vi "NumIntegrate_Rkf45impl_Ax_Bu_K.vi"(4 "MaxTruncError":dbl, 5 "A":T1, 6 "dT_Remaining":dbl, 7 "B":T1, 8 "InitialH":dbl, 9 "K":T1, 10 "U":T1, 11 "X":T1) -> (1 "IterationCount":i32, 2 "H":dbl, 3 "NewX":T1)   [LabVIEW 2019, in "Trajectory_Library.lvlib"]
doc: "Creates a new LINEAR SYSTEM data cluster with the specified values. \n\n\nInputs: \n - XXX -- XXX.\n\nOutputs:\n - XXX -- XXX."
uses:
  Trajectory_Library.lvlib
  <vilib>/Analysis/Matrix/Datatypes/RealMatrix.ctl
  <vilib>/Analysis/_algsub.llb/Matrix Norm Type.ctl
  <vilib>/Analysis/_algsub.llb/Real Matrix Norm.vi
  <vilib>/Analysis/Matrix/Numeric/Multiply/Multiply - RM,R.vi
  <vilib>/Analysis/Matrix/Numeric/Add/Add - RM,RM.vi
  <vilib>/Analysis/Matrix/NI_Matrix.lvlib
  <vilib>/Analysis/NI_AALPro.lvlib
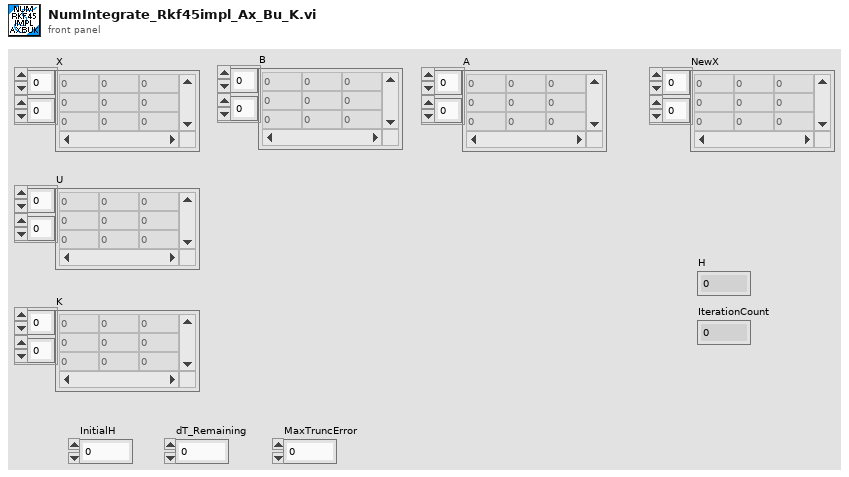
[diagram p1: front panel]
types:
  T1 = typedef "NI_Matrix.lvlib/RealMatrix.ctl" = dbl[][]
  T2 = typedef "NI_AALPro.lvlib/Matrix Norm Type.ctl" = i32
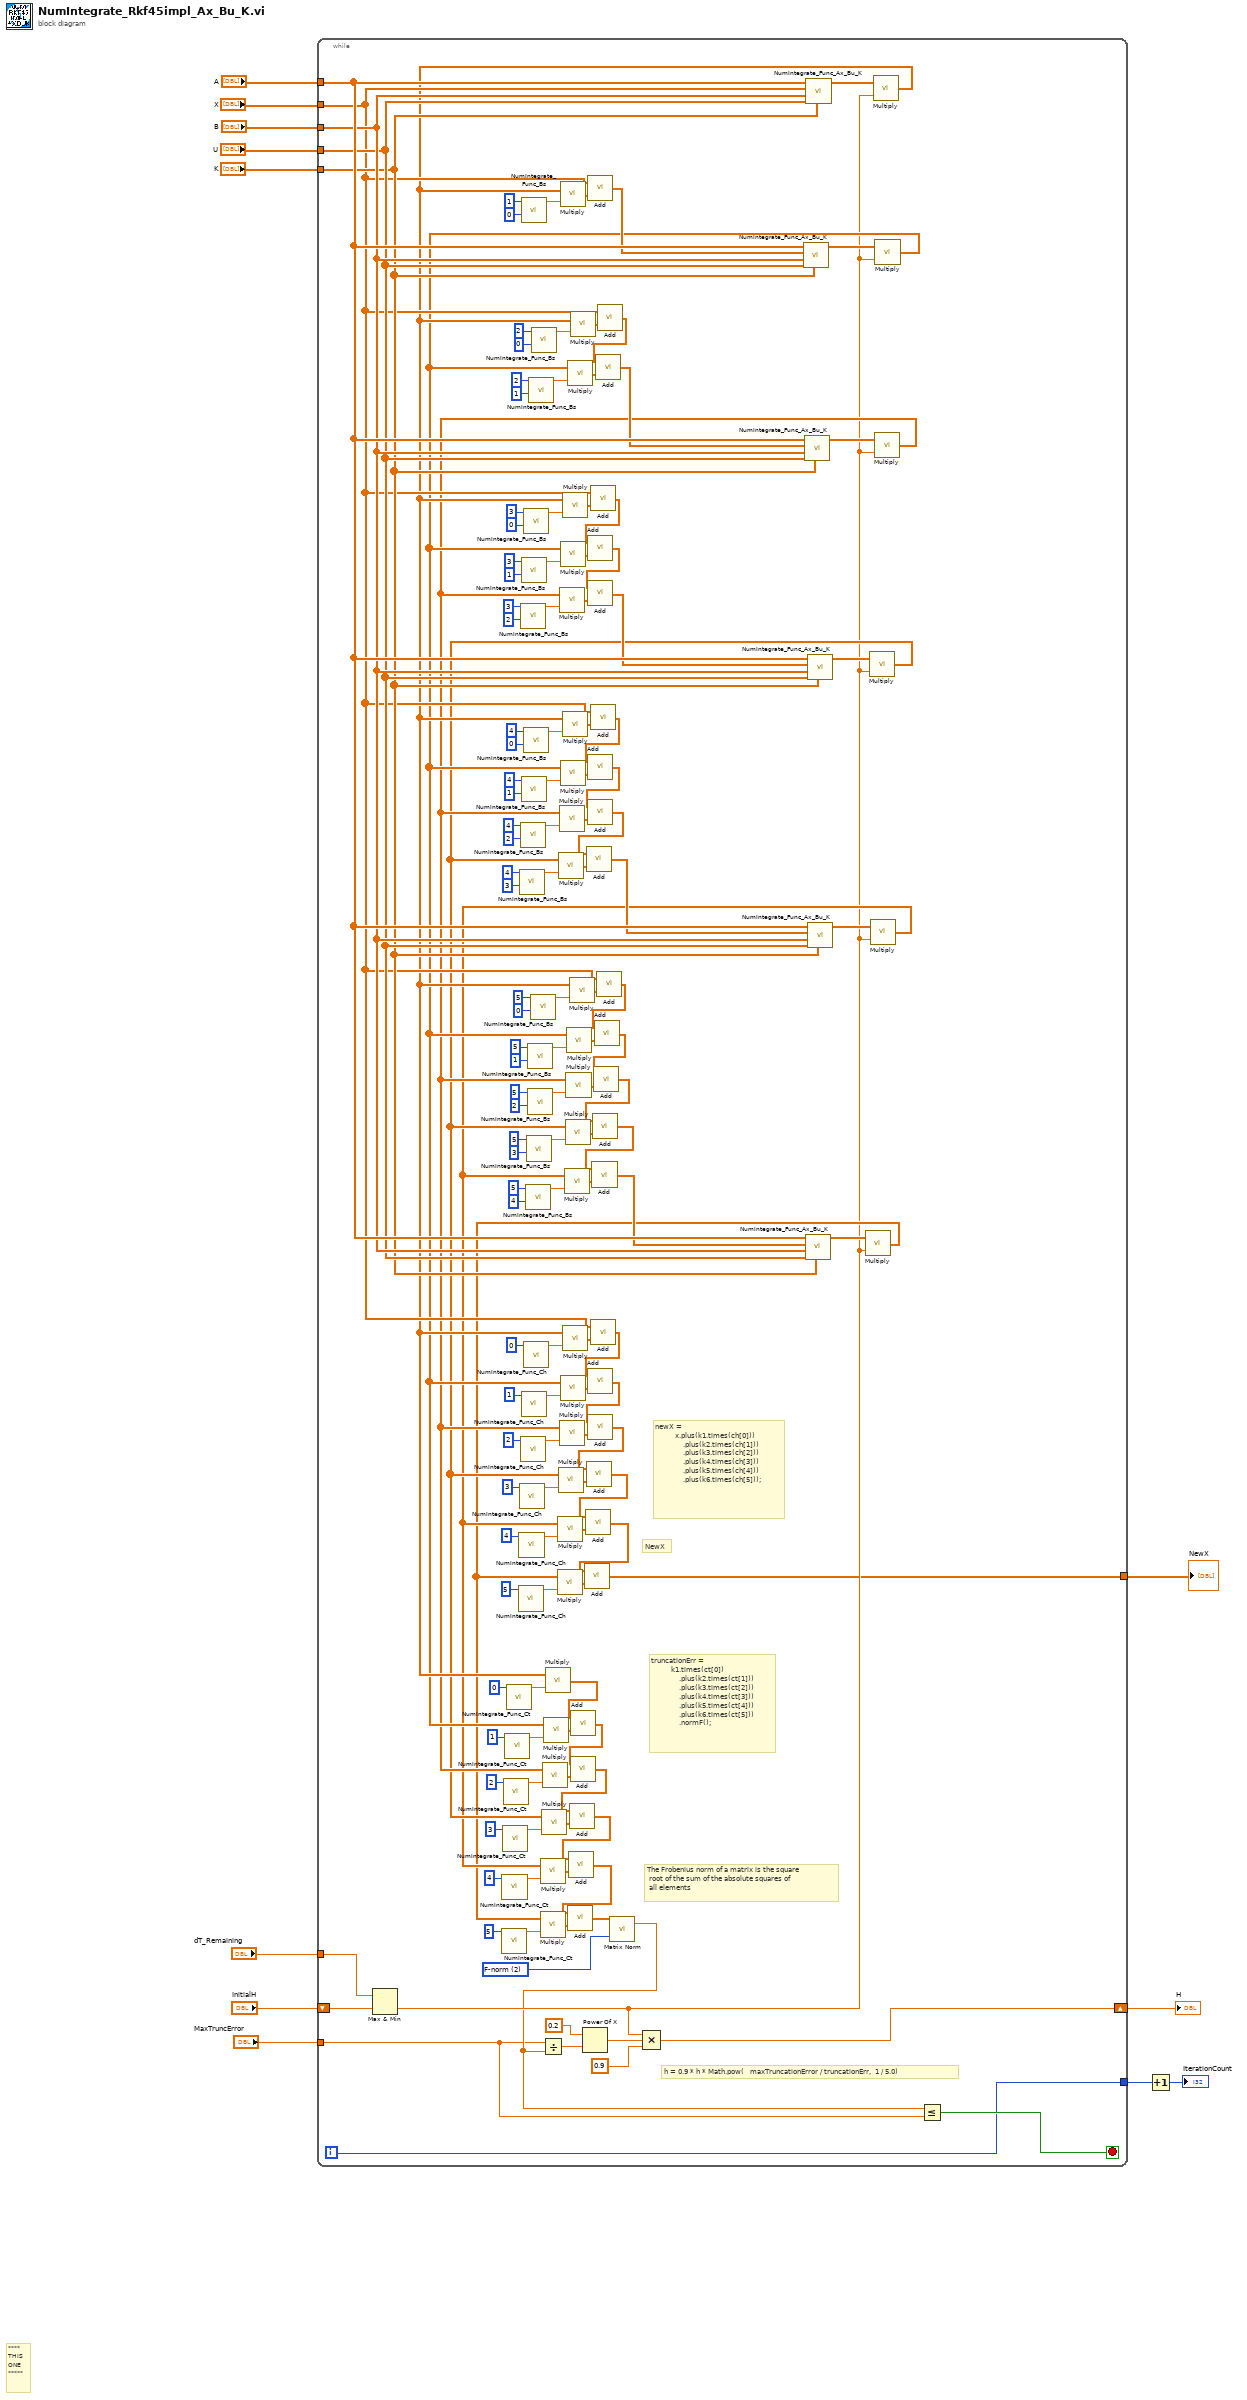
[diagram p0: block diagram]
diagram:
  # "****\nTHIS\nONE\n*****"
  n1 = while {
    tunnel: "A" -> [w164]
    tunnel: "B" -> [w162]
    tunnel: "K" -> [w160]
    shift-right: [w21] -> w4
    shift-left: "InitialH" -> [w20]
    tunnel: "X" -> [w60]
    tunnel: "U" -> [w161]
    tunnel: "MaxTruncError" -> [w16]
    tunnel: "dT_Remaining" -> [w19]
    tunnel: [w14] -> w1
    tunnel: [w13] -> w3
    i -> [w13]
    stop <- w15 stop-if-true
    w26 = T2 2 items=["2-norm", "1-norm", "F-norm", "Inf-norm"] ("norm type")
    # "h = 0.9 * h * Math.pow(   maxTruncationError / truncationErr,  1 / 5.0)"
    # "The Frobenius norm of a matrix is the square\n root of the sum of the absolute squares of\n all elements"
    # "truncationErr =\n          k1.times(ct[0])\n              .plus(k2.times(ct[1]))\n              .plus(k3.times(ct[2]))\n              .plus(k4.times(ct[3]))\n              .plus(k5.times(ct[4]))\n              .plus(k6.times(ct[5]))\n              .normF();"
    # "NewX"
    # "newX =\n          x.plus(k1.times(ch[0]))\n              .plus(k2.times(ch[1]))\n              .plus(k3.times(ch[2]))\n              .plus(k4.times(ch[3]))\n              .plus(k5.times(ch[4]))\n              .plus(k6.times(ch[5]));"
    n2 = Max & Min(x=w19, y=w20) -> (min(x,y)=w18:dbl)  [unwired: 1 out]
    n3 = call "NumIntegrate_Func_Ct.vi"("Index"=5 ("Row")) -> ("Ct"=w38:dbl)  [unwired: 10 in]
    n4 = call "NumIntegrate_Func_Ct.vi"("Index"=4 ("Row")) -> ("Ct"=w42:dbl)  [unwired: 10 in]
    n5 = call "NumIntegrate_Func_Ct.vi"("Index"=3 ("Row")) -> ("Ct"=w46:dbl)  [unwired: 10 in]
    n6 = call "NumIntegrate_Func_Ct.vi"("Index"=2 ("Row")) -> ("Ct"=w50:dbl)  [unwired: 10 in]
    n7 = call "NumIntegrate_Func_Ct.vi"("Index"=1 ("Row")) -> ("Ct"=w53:dbl)  [unwired: 10 in]
    n8 = call "NumIntegrate_Func_Ct.vi"("Index"=0 ("Row")) -> ("Ct"=w55:dbl)  [unwired: 10 in]
    n9 = call "NumIntegrate_Func_Ch.vi"("Index"=5 ("Row")) -> ("Ch"=w59:dbl)  [unwired: 10 in]
    n10 = call "NumIntegrate_Func_Ch.vi"("Index"=4 ("Row")) -> ("Ch"=w64:dbl)  [unwired: 10 in]
    n11 = call "NumIntegrate_Func_Bs.vi"("Col"=3, "Row"=4) -> ("Bs"=w110:dbl)  [unwired: 9 in]
    n12 = call "NumIntegrate_Func_Ch.vi"("Index"=3 ("Row")) -> ("Ch"=w68:dbl)  [unwired: 10 in]
    n13 = call "NumIntegrate_Func_Bs.vi"("Col"=2, "Row"=3) -> ("Bs"=w130:dbl)  [unwired: 9 in]
    n14 = call "NumIntegrate_Func_Bs.vi"("Col"=2, "Row"=4) -> ("Bs"=w115:dbl)  [unwired: 9 in]
    n15 = call "NumIntegrate_Func_Ch.vi"("Index"=2 ("Row")) -> ("Ch"=w72:dbl)  [unwired: 10 in]
    n16 = call "NumIntegrate_Func_Bs.vi"("Col"=0, "Row"=1) -> ("Bs"=w154:dbl)  [unwired: 9 in]
    n17 = call "NumIntegrate_Func_Bs.vi"("Col"=1, "Row"=3) -> ("Bs"=w135:dbl)  [unwired: 9 in]
    n18 = call "NumIntegrate_Func_Bs.vi"("Col"=1, "Row"=4) -> ("Bs"=w120:dbl)  [unwired: 9 in]
    n19 = call "NumIntegrate_Func_Ch.vi"("Index"=1 ("Row")) -> ("Ch"=w76:dbl)  [unwired: 10 in]
    n20 = call "NumIntegrate_Func_Bs.vi"("Col"=0, "Row"=3) -> ("Bs"=w139:dbl)  [unwired: 9 in]
    n21 = call "NumIntegrate_Func_Bs.vi"("Col"=0, "Row"=4) -> ("Bs"=w124:dbl)  [unwired: 9 in]
    n22 = call "NumIntegrate_Func_Ch.vi"("Index"=0 ("Row")) -> ("Ch"=w79:dbl)  [unwired: 10 in]
    n23 = call "NumIntegrate_Func_Bs.vi"("Col"=4, "Row"=5) -> ("Bs"=w85:dbl)  [unwired: 9 in]
    n24 = call "NumIntegrate_Func_Bs.vi"("Col"=3, "Row"=5) -> ("Bs"=w90:dbl)  [unwired: 9 in]
    n25 = call "NumIntegrate_Func_Bs.vi"("Col"=2, "Row"=5) -> ("Bs"=w95:dbl)  [unwired: 9 in]
    n26 = call "NumIntegrate_Func_Bs.vi"("Col"=1, "Row"=5) -> ("Bs"=w100:dbl)  [unwired: 9 in]
    n27 = call "NumIntegrate_Func_Bs.vi"("Col"=1, "Row"=2) -> ("Bs"=w145:dbl)  [unwired: 9 in]
    n28 = call "NumIntegrate_Func_Bs.vi"("Col"=0, "Row"=5) -> ("Bs"=w104:dbl)  [unwired: 9 in]
    n29 = call "NumIntegrate_Func_Bs.vi"("Col"=0, "Row"=2) -> ("Bs"=w149:dbl)  [unwired: 9 in]
    n30 = call "NumIntegrate_Func_Ax_Bu_K.vi"("K"=w160, "U"=w161, "B"=w162, "X"=w60, "A"=w164) -> ("output matrix"=w163:T1)  [unwired: 5 in, 1 out]
    n31 = call-poly <vilib>:"Multiply.vi"("Real Scalar c"=w18, "Real Matrix A"=w163) -> ("A * c"=w34:T1)
    n32 = call-poly <vilib>:"Multiply.vi"("Real Scalar c"=w55, "Real Matrix A"=w34) -> ("A * c"=w33:T1)
    n33 = call-poly <vilib>:"Multiply.vi"("Real Scalar c"=w154, "Real Matrix A"=w34) -> ("A * c"=w153:T1)
    n34 = call-poly <vilib>:"Multiply.vi"("Real Scalar c"=w139, "Real Matrix A"=w34) -> ("A * c"=w138:T1)
    n35 = call-poly <vilib>:"Multiply.vi"("Real Scalar c"=w124, "Real Matrix A"=w34) -> ("A * c"=w123:T1)
    n36 = call-poly <vilib>:"Multiply.vi"("Real Scalar c"=w79, "Real Matrix A"=w34) -> ("A * c"=w78:T1)
    n37 = call-poly <vilib>:"Multiply.vi"("Real Scalar c"=w104, "Real Matrix A"=w34) -> ("A * c"=w103:T1)
    n38 = call-poly <vilib>:"Multiply.vi"("Real Scalar c"=w149, "Real Matrix A"=w34) -> ("A * c"=w148:T1)
    n39 = call-poly <vilib>:"Add.vi"("Real Matrix B"=w153, "Real Matrix A"=w60) -> ("A + B"=w152:T1)
    n40 = call-poly <vilib>:"Add.vi"("Real Matrix B"=w138, "Real Matrix A"=w60) -> ("A + B"=w131:T1)
    n41 = call-poly <vilib>:"Add.vi"("Real Matrix B"=w123, "Real Matrix A"=w60) -> ("A + B"=w116:T1)
    n42 = call-poly <vilib>:"Add.vi"("Real Matrix B"=w78, "Real Matrix A"=w60) -> ("A + B"=w73:T1)
    n43 = call-poly <vilib>:"Add.vi"("Real Matrix B"=w103, "Real Matrix A"=w60) -> ("A + B"=w96:T1)
    n44 = call-poly <vilib>:"Add.vi"("Real Matrix B"=w148, "Real Matrix A"=w60) -> ("A + B"=w141:T1)
    n45 = call "NumIntegrate_Func_Ax_Bu_K.vi"("K"=w160, "U"=w161, "B"=w162, "X"=w152, "A"=w164) -> ("output matrix"=w155:T1)  [unwired: 5 in, 1 out]
    n46 = call-poly <vilib>:"Multiply.vi"("Real Scalar c"=w18, "Real Matrix A"=w155) -> ("A * c"=w32:T1)
    n47 = call-poly <vilib>:"Multiply.vi"("Real Scalar c"=w53, "Real Matrix A"=w32) -> ("A * c"=w52:T1)
    n48 = call-poly <vilib>:"Multiply.vi"("Real Scalar c"=w135, "Real Matrix A"=w32) -> ("A * c"=w134:T1)
    n49 = call-poly <vilib>:"Multiply.vi"("Real Scalar c"=w120, "Real Matrix A"=w32) -> ("A * c"=w119:T1)
    n50 = call-poly <vilib>:"Multiply.vi"("Real Scalar c"=w76, "Real Matrix A"=w32) -> ("A * c"=w75:T1)
    n51 = call-poly <vilib>:"Multiply.vi"("Real Scalar c"=w100, "Real Matrix A"=w32) -> ("A * c"=w99:T1)
    n52 = call-poly <vilib>:"Multiply.vi"("Real Scalar c"=w145, "Real Matrix A"=w32) -> ("A * c"=w144:T1)
    n53 = call-poly <vilib>:"Add.vi"("Real Matrix B"=w52, "Real Matrix A"=w33) -> ("A + B"=w47:T1)
    n54 = call-poly <vilib>:"Add.vi"("Real Matrix B"=w134, "Real Matrix A"=w131) -> ("A + B"=w126:T1)
    n55 = call-poly <vilib>:"Add.vi"("Real Matrix B"=w119, "Real Matrix A"=w116) -> ("A + B"=w111:T1)
    n56 = call-poly <vilib>:"Add.vi"("Real Matrix B"=w75, "Real Matrix A"=w73) -> ("A + B"=w69:T1)
    n57 = call-poly <vilib>:"Add.vi"("Real Matrix B"=w99, "Real Matrix A"=w96) -> ("A + B"=w91:T1)
    n58 = call-poly <vilib>:"Add.vi"("Real Matrix B"=w144, "Real Matrix A"=w141) -> ("A + B"=w140:T1)
    n59 = call "NumIntegrate_Func_Ax_Bu_K.vi"("K"=w160, "U"=w161, "B"=w162, "X"=w140, "A"=w164) -> ("output matrix"=w156:T1)  [unwired: 5 in, 1 out]
    n60 = call-poly <vilib>:"Multiply.vi"("Real Scalar c"=w18, "Real Matrix A"=w156) -> ("A * c"=w31:T1)
    n61 = call-poly <vilib>:"Multiply.vi"("Real Scalar c"=w50, "Real Matrix A"=w31) -> ("A * c"=w49:T1)
    n62 = call-poly <vilib>:"Multiply.vi"("Real Scalar c"=w130, "Real Matrix A"=w31) -> ("A * c"=w129:T1)
    n63 = call-poly <vilib>:"Multiply.vi"("Real Scalar c"=w115, "Real Matrix A"=w31) -> ("A * c"=w114:T1)
    n64 = call-poly <vilib>:"Multiply.vi"("Real Scalar c"=w72, "Real Matrix A"=w31) -> ("A * c"=w71:T1)
    n65 = call-poly <vilib>:"Multiply.vi"("Real Scalar c"=w95, "Real Matrix A"=w31) -> ("A * c"=w94:T1)
    n66 = call-poly <vilib>:"Add.vi"("Real Matrix B"=w49, "Real Matrix A"=w47) -> ("A + B"=w43:T1)
    n67 = call-poly <vilib>:"Add.vi"("Real Matrix B"=w129, "Real Matrix A"=w126) -> ("A + B"=w125:T1)
    n68 = call-poly <vilib>:"Add.vi"("Real Matrix B"=w114, "Real Matrix A"=w111) -> ("A + B"=w106:T1)
    n69 = call-poly <vilib>:"Add.vi"("Real Matrix B"=w71, "Real Matrix A"=w69) -> ("A + B"=w65:T1)
    n70 = call-poly <vilib>:"Add.vi"("Real Matrix B"=w94, "Real Matrix A"=w91) -> ("A + B"=w86:T1)
    n71 = call "NumIntegrate_Func_Ax_Bu_K.vi"("K"=w160, "U"=w161, "B"=w162, "X"=w125, "A"=w164) -> ("output matrix"=w157:T1)  [unwired: 5 in, 1 out]
    n72 = call-poly <vilib>:"Multiply.vi"("Real Scalar c"=w18, "Real Matrix A"=w157) -> ("A * c"=w30:T1)
    n73 = call-poly <vilib>:"Multiply.vi"("Real Scalar c"=w46, "Real Matrix A"=w30) -> ("A * c"=w45:T1)
    n74 = call-poly <vilib>:"Multiply.vi"("Real Scalar c"=w110, "Real Matrix A"=w30) -> ("A * c"=w109:T1)
    n75 = call-poly <vilib>:"Multiply.vi"("Real Scalar c"=w68, "Real Matrix A"=w30) -> ("A * c"=w67:T1)
    n76 = call-poly <vilib>:"Multiply.vi"("Real Scalar c"=w90, "Real Matrix A"=w30) -> ("A * c"=w89:T1)
    n77 = call-poly <vilib>:"Add.vi"("Real Matrix B"=w45, "Real Matrix A"=w43) -> ("A + B"=w39:T1)
    n78 = call-poly <vilib>:"Add.vi"("Real Matrix B"=w109, "Real Matrix A"=w106) -> ("A + B"=w105:T1)
    n79 = call-poly <vilib>:"Add.vi"("Real Matrix B"=w67, "Real Matrix A"=w65) -> ("A + B"=w61:T1)
    n80 = call-poly <vilib>:"Add.vi"("Real Matrix B"=w89, "Real Matrix A"=w86) -> ("A + B"=w81:T1)
    n81 = call "NumIntegrate_Func_Ax_Bu_K.vi"("K"=w160, "U"=w161, "B"=w162, "X"=w105, "A"=w164) -> ("output matrix"=w158:T1)  [unwired: 5 in, 1 out]
    n82 = call-poly <vilib>:"Multiply.vi"("Real Scalar c"=w18, "Real Matrix A"=w158) -> ("A * c"=w29:T1)
    n83 = call-poly <vilib>:"Multiply.vi"("Real Scalar c"=w42, "Real Matrix A"=w29) -> ("A * c"=w41:T1)
    n84 = call-poly <vilib>:"Multiply.vi"("Real Scalar c"=w64, "Real Matrix A"=w29) -> ("A * c"=w63:T1)
    n85 = call-poly <vilib>:"Multiply.vi"("Real Scalar c"=w85, "Real Matrix A"=w29) -> ("A * c"=w84:T1)
    n86 = call-poly <vilib>:"Add.vi"("Real Matrix B"=w41, "Real Matrix A"=w39) -> ("A + B"=w35:T1)
    n87 = call-poly <vilib>:"Add.vi"("Real Matrix B"=w63, "Real Matrix A"=w61) -> ("A + B"=w56:T1)
    n88 = call-poly <vilib>:"Add.vi"("Real Matrix B"=w84, "Real Matrix A"=w81) -> ("A + B"=w80:T1)
    n89 = call "NumIntegrate_Func_Ax_Bu_K.vi"("K"=w160, "U"=w161, "B"=w162, "X"=w80, "A"=w164) -> ("output matrix"=w159:T1)  [unwired: 5 in, 1 out]
    n90 = call-poly <vilib>:"Multiply.vi"("Real Scalar c"=w18, "Real Matrix A"=w159) -> ("A * c"=w28:T1)
    n91 = call-poly <vilib>:"Multiply.vi"("Real Scalar c"=w38, "Real Matrix A"=w28) -> ("A * c"=w37:T1)
    n92 = call-poly <vilib>:"Multiply.vi"("Real Scalar c"=w59, "Real Matrix A"=w28) -> ("A * c"=w58:T1)
    n93 = call-poly <vilib>:"Add.vi"("Real Matrix B"=w37, "Real Matrix A"=w35) -> ("A + B"=w27:T1)
    n94 = call-poly <vilib>:"Add.vi"("Real Matrix B"=w58, "Real Matrix A"=w56) -> ("A + B"=w14:T1)
    n95 = call-poly <vilib>:"Matrix Norm.vi"("norm type"=w26, "Input Matrix"=w27) -> ("norm"=w17:dbl)  [unwired: 1 out]
    n96 = Divide(x=w16, y=w17) -> (x/y=w24:dbl)
    n97 = Power Of X(1:w24, 2:0.2 ("x")) -> (0:w23:dbl)
    n98 = Compound Arithmetic op=MULTIPLY(w18, w23, 0.9 ("value")) -> (w21:dbl)
    n99 = Less Or Equal?(x=w17, y=w16) -> (x <= y?=w15:bool)
  }
  "NewX" <- w1
  "H" <- w4
  n100 = Increment(x=w3) -> (x+1=→"IterationCount":i32)
